vi "PI_Controller.vi"(0 "SP":dbl, 1 "Init":bool, 5 "PV":dbl, 7 "A":dbl, 9 "T0":dbl, 11 "dt":dbl, 12 "U min":dbl, 13 "U max":dbl) -> (4 "U out":dbl)   [LabVIEW 2019]
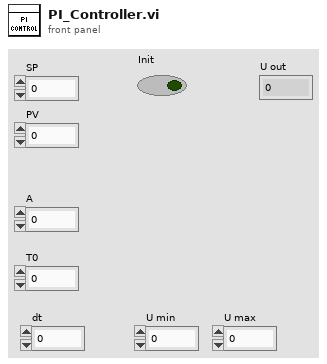
[diagram p1: front panel]
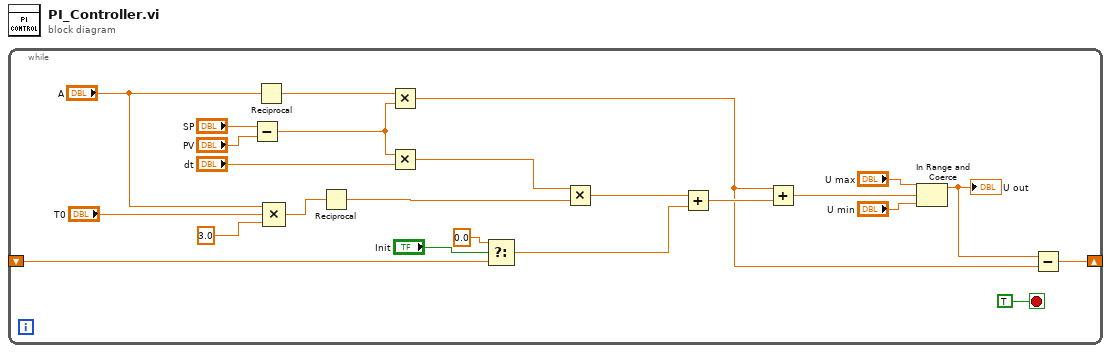
[diagram p0: block diagram]
diagram:
  n1 = while {
    shift-right: [w7] -> _
    shift-left: _ -> [w4]
    stop <- TRUE stop-if-true
    n2 = Subtract(x="SP", y="PV") -> (x-y=w18:dbl)
    n3 = Reciprocal(x="A") -> (1/x=w24:dbl)
    n4 = Compound Arithmetic op=MULTIPLY("A", "T0", 3.0 ("y")) -> (w21:dbl)
    n5 = Reciprocal(x=w21) -> (1/x=w16:dbl)
    n6 = Multiply(x=w24, y=w18) -> (x*y=w8:dbl)
    n7 = Multiply(x=w18, y="dt") -> (x*y=w12:dbl)
    n8 = Select(t=0.0, s="Init", f=w4) -> (s? t:f=w5:dbl)
    n9 = Multiply(x=w12, y=w16) -> (x*y=w11:dbl)
    n10 = Add(x=w11, y=w5) -> (x+y=w10:dbl)
    n11 = Add(x=w8, y=w10) -> (x+y=w9:dbl)
    n12 = In Range and Coerce(upper limit="U max", x=w9, lower limit="U min") -> (coerced(x)=w6:dbl)  [unwired: 1 out]
    "U out" <- w6
    n13 = Subtract(x=w6, y=w8) -> (x-y=w7:dbl)
  }
